vi "daqtest.vi"() -> ()   [LabVIEW 2020]
uses:
  <vilib>/DAQmx/write.llb/DAQmx Write (Analog DBL 1Chan 1Samp).vi
  <vilib>/DAQmx/write.llb/DAQmx Write (Digital Bool 1Line 1Point).vi
  <vilib>/DAQmx/create/channels.llb/DAQmx Create Channel (DO-Digital Output).vi
  <vilib>/DAQmx/miscellaneous.llb/DAQmx Fill In Error Info.vi
  <vilib>/DAQmx/create/channels.llb/DAQmx Create Channel (AO-Voltage-Basic).vi
panel:
  in  "Blanking channel":tag="Dev1/ao0"
  in  "stop":bool
  in  "physical channels 4":tag
  in  "physical channels 2":tag
  in  "physical channels":tag
  in  "Laser Channel 3":tag
  in  "Vmode":dbl=5.0 min=0.0 max=5.0
  in  "Digital Blanking Channel":tag="Dev1/port0/line4"
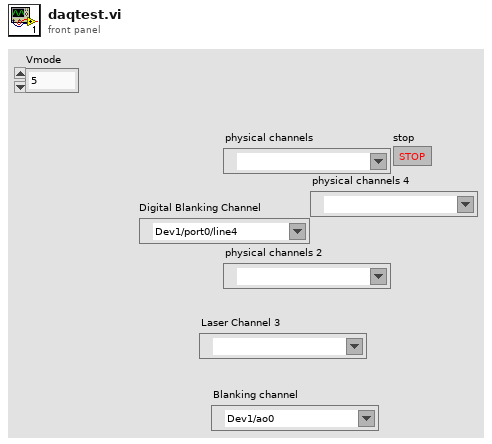
[diagram p1: front panel]
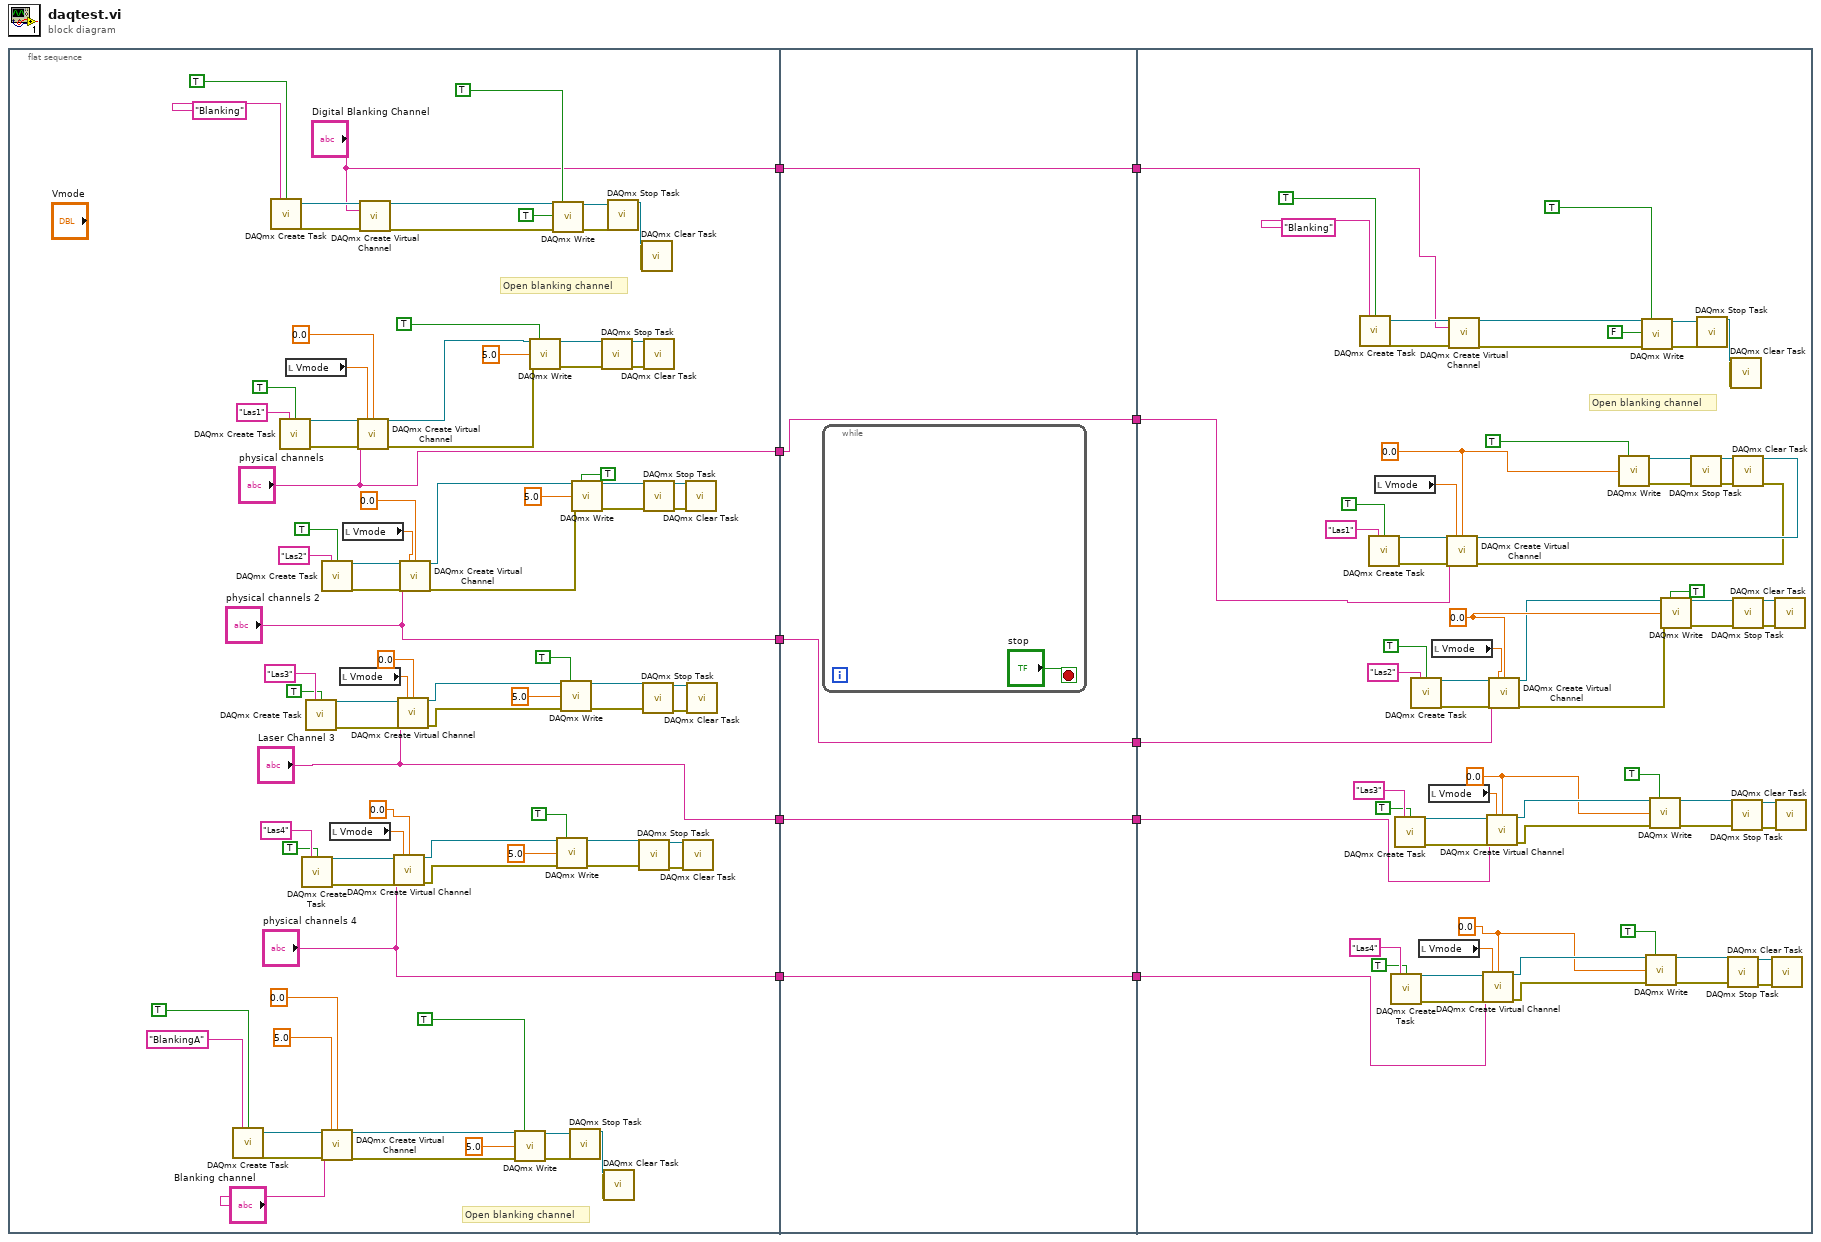
[diagram p0: block diagram]
diagram:
  n1 = flat-sequence {
    tunnel: ["Laser Channel 3"] -> w9
    tunnel: ["physical channels 4"] -> w7
    tunnel: ["physical channels 2"] -> w6
    tunnel: ["physical channels"] -> w3
    tunnel: ["Digital Blanking Channel"] -> w2
    tunnel: [w103] -> w10
    tunnel: w9 -> [w103]
    tunnel: [w102] -> w8
    tunnel: w7 -> [w102]
    tunnel: w6 -> [w101]
    tunnel: [w101] -> w5
    tunnel: [w100] -> w4
    tunnel: w3 -> [w100]
    tunnel: w2 -> [w99]
    tunnel: [w99] -> w1
    tunnel: w10 -> [w109]
    tunnel: w8 -> [w108]
    tunnel: w5 -> [w107]
    tunnel: w4 -> [w106]
    tunnel: w1 -> [w105]
    frame #0 {
      # "Open blanking channel"
      # "Open blanking channel"
      n2 = call <vilib>:"DAQmx Create Task.vi"("new task name"="BlankingA", "auto cleanup"=TRUE) -> ("task out"=w22:refnum<k21>, "error out"=w23:errorcluster)  [unwired: 12 in]
      n3 = call <vilib>:"DAQmx Create Task.vi"("new task name"="Blanking", "auto cleanup"=TRUE) -> ("task out"=w95:refnum<k21>, "error out"=w96:errorcluster)  [unwired: 12 in]
      n4 = call <vilib>:"DAQmx Create Task.vi"("new task name"="Las1", "auto cleanup"=TRUE) -> ("task out"=w68:refnum<k21>, "error out"=w67:errorcluster)  [unwired: 12 in]
      n5 = local read "Vmode"() -> (w64:dbl)
      n6 = call <vilib>:"DAQmx Create Task.vi"("new task name"="Las4", "auto cleanup"=TRUE) -> ("task out"=w48:refnum<k21>, "error out"=w46:errorcluster)  [unwired: 12 in]
      n7 = call <vilib>:"DAQmx Create Task.vi"("new task name"="Las3", "auto cleanup"=TRUE) -> ("task out"=w61:refnum<k21>, "error out"=w58:errorcluster)  [unwired: 12 in]
      n8 = call <vilib>:"DAQmx Create Task.vi"("new task name"="Las2", "auto cleanup"=TRUE) -> ("task out"=w80:refnum<k21>, "error out"=w79:errorcluster)  [unwired: 12 in]
      n9 = call-poly <vilib>:"DAQmx Create Virtual Channel.vi"("task in"=w22, "maximum value"=5.0, "minimum value"=0.0, "physical channels"="Blanking channel", "error in"=w23) -> ("task out"=w21:refnum<k21>, "error out"=w20:errorcluster)  [unwired: 9 in]
      n10 = local read "Vmode"() -> (w38:dbl)
      n11 = local read "Vmode"() -> (w60:dbl)
      n12 = local read "Vmode"() -> (w63:dbl)
      n13 = call-poly <vilib>:"DAQmx Create Virtual Channel.vi"("task in"=w68, "maximum value"=w64, "minimum value"=0.0 ("data"), "physical channels"="physical channels", "error in"=w67) -> ("task out"=w27:refnum<k21>, "error out"=w26:errorcluster)  [unwired: 9 in]
      n14 = call-poly <vilib>:"DAQmx Create Virtual Channel.vi"("task in"=w95, "lines"="Digital Blanking Channel", "error in"=w96) -> ("task out"=w94:refnum<k21>, "error out"=w93:errorcluster)  [unwired: 11 in]
      n15 = call-poly <vilib>:"DAQmx Create Virtual Channel.vi"("task in"=w48, "maximum value"=w38, "minimum value"=0.0, "physical channels"="physical channels 4", "error in"=w46) -> ("task out"=w45:refnum<k21>, "error out"=w44:errorcluster)  [unwired: 9 in]
      n16 = call-poly <vilib>:"DAQmx Create Virtual Channel.vi"("task in"=w61, "maximum value"=w60, "minimum value"=0.0, "physical channels"="Laser Channel 3", "error in"=w58) -> ("task out"=w57:refnum<k21>, "error out"=w56:errorcluster)  [unwired: 9 in]
      n17 = call-poly <vilib>:"DAQmx Create Virtual Channel.vi"("task in"=w80, "maximum value"=w63, "minimum value"=0.0 ("data"), "physical channels"="physical channels 2", "error in"=w79) -> ("task out"=w78:refnum<k21>, "error out"=w77:errorcluster)  [unwired: 9 in]
      n18 = call-poly <vilib>:"DAQmx Write.vi"("task/channels in"=w21, "auto start"=TRUE, "data"=5.0, "error in"=w20) -> ("task out"=w25:refnum<k21>, "error out"=w24:errorcluster)  [unwired: 9 in, 1 out]
      n19 = call-poly <vilib>:"DAQmx Write.vi"("task/channels in"=w27, "auto start"=TRUE ("auto cleanup"), "data"=5.0, "error in"=w26) -> ("task out"=w70:refnum<k21>, "error out"=w69:errorcluster)  [unwired: 9 in, 1 out]
      n20 = call-poly <vilib>:"DAQmx Write.vi"("task/channels in"=w94, "auto start"=TRUE, "data"=TRUE, "error in"=w93) -> ("task out"=w98:refnum<k21>, "error out"=w97:errorcluster)  [unwired: 9 in, 1 out]
      n21 = call-poly <vilib>:"DAQmx Write.vi"("task/channels in"=w45, "auto start"=TRUE, "data"=5.0, "error in"=w44) -> ("task out"=w40:refnum<k21>, "error out"=w39:errorcluster)  [unwired: 9 in, 1 out]
      n22 = call-poly <vilib>:"DAQmx Write.vi"("task/channels in"=w57, "auto start"=TRUE, "data"=5.0, "error in"=w56) -> ("task out"=w51:refnum<k21>, "error out"=w50:errorcluster)  [unwired: 9 in, 1 out]
      n23 = call <vilib>:"DAQmx Stop Task.vi"("task/channels in"=w25, "error in"=w24) -> ("task out"=w18:refnum<k21>, "error out"=w17:errorcluster)  [unwired: 12 in]
      n24 = call-poly <vilib>:"DAQmx Write.vi"("task/channels in"=w78, "auto start"=TRUE ("auto cleanup"), "data"=5.0, "error in"=w77) -> ("task out"=w82:refnum<k21>, "error out"=w81:errorcluster)  [unwired: 9 in, 1 out]
      n25 = call <vilib>:"DAQmx Stop Task.vi"("task/channels in"=w70, "error in"=w69) -> ("task out"=w66:refnum<k21>, "error out"=w65:errorcluster)  [unwired: 12 in]
      n26 = call <vilib>:"DAQmx Clear Task.vi"("task in"=w18, "error in"=w17) -> ()  [unwired: 13 in, 1 out]
      n27 = call <vilib>:"DAQmx Stop Task.vi"("task/channels in"=w98, "error in"=w97) -> ("task out"=w91:refnum<k21>, "error out"=w90:errorcluster)  [unwired: 12 in]
      n28 = call <vilib>:"DAQmx Stop Task.vi"("task/channels in"=w40, "error in"=w39) -> ("task out"=w42:refnum<k21>, "error out"=w41:errorcluster)  [unwired: 12 in]
      n29 = call <vilib>:"DAQmx Clear Task.vi"("task in"=w91, "error in"=w90) -> ()  [unwired: 13 in, 1 out]
      n30 = call <vilib>:"DAQmx Stop Task.vi"("task/channels in"=w51, "error in"=w50) -> ("task out"=w53:refnum<k21>, "error out"=w52:errorcluster)  [unwired: 12 in]
      n31 = call <vilib>:"DAQmx Clear Task.vi"("task in"=w66, "error in"=w65) -> ()  [unwired: 13 in, 1 out]
      n32 = call <vilib>:"DAQmx Stop Task.vi"("task/channels in"=w82, "error in"=w81) -> ("task out"=w76:refnum<k21>, "error out"=w75:errorcluster)  [unwired: 12 in]
      n33 = call <vilib>:"DAQmx Clear Task.vi"("task in"=w42, "error in"=w41) -> ()  [unwired: 13 in, 1 out]
      n34 = call <vilib>:"DAQmx Clear Task.vi"("task in"=w76, "error in"=w75) -> ()  [unwired: 13 in, 1 out]
      n35 = call <vilib>:"DAQmx Clear Task.vi"("task in"=w53, "error in"=w52) -> ()  [unwired: 13 in, 1 out]
    }
    frame #1 {
      n36 = while {
        stop <- "stop" stop-if-true
      }
    }
    frame #2 {
      w110 = 0.0 ("minimum value")
      w127 = 0.0 ("minimum value")
      w161 = 0.0 ("data")
      w149 = 0.0 ("data")
      # "Open blanking channel"
      n37 = call <vilib>:"DAQmx Create Task.vi"("new task name"="Blanking", "auto cleanup"=TRUE) -> ("task out"=w170:refnum<k21>, "error out"=w171:errorcluster)  [unwired: 12 in]
      n38 = call <vilib>:"DAQmx Create Task.vi"("new task name"="Las1", "auto cleanup"=TRUE) -> ("task out"=w143:refnum<k21>, "error out"=w142:errorcluster)  [unwired: 12 in]
      n39 = local read "Vmode"() -> (w137:dbl)
      n40 = call <vilib>:"DAQmx Create Task.vi"("new task name"="Las4", "auto cleanup"=TRUE) -> ("task out"=w121:refnum<k21>, "error out"=w119:errorcluster)  [unwired: 12 in]
      n41 = call <vilib>:"DAQmx Create Task.vi"("new task name"="Las3", "auto cleanup"=TRUE) -> ("task out"=w134:refnum<k21>, "error out"=w131:errorcluster)  [unwired: 12 in]
      n42 = call <vilib>:"DAQmx Create Task.vi"("new task name"="Las2", "auto cleanup"=TRUE) -> ("task out"=w155:refnum<k21>, "error out"=w154:errorcluster)  [unwired: 12 in]
      n43 = local read "Vmode"() -> (w111:dbl)
      n44 = local read "Vmode"() -> (w133:dbl)
      n45 = local read "Vmode"() -> (w136:dbl)
      n46 = call-poly <vilib>:"DAQmx Create Virtual Channel.vi"("task in"=w143, "maximum value"=w137, "minimum value"=w149, "physical channels"=w106, "error in"=w142) -> ("task out"=w141:refnum<k21>, "error out"=w140:errorcluster)  [unwired: 9 in]
      n47 = call-poly <vilib>:"DAQmx Create Virtual Channel.vi"("task in"=w170, "lines"=w105, "error in"=w171) -> ("task out"=w169:refnum<k21>, "error out"=w168:errorcluster)  [unwired: 11 in]
      n48 = call-poly <vilib>:"DAQmx Create Virtual Channel.vi"("task in"=w121, "maximum value"=w111, "minimum value"=w110, "physical channels"=w108, "error in"=w119) -> ("task out"=w118:refnum<k21>, "error out"=w117:errorcluster)  [unwired: 9 in]
      n49 = call-poly <vilib>:"DAQmx Create Virtual Channel.vi"("task in"=w134, "maximum value"=w133, "minimum value"=w127, "physical channels"=w109, "error in"=w131) -> ("task out"=w130:refnum<k21>, "error out"=w129:errorcluster)  [unwired: 9 in]
      n50 = call-poly <vilib>:"DAQmx Create Virtual Channel.vi"("task in"=w155, "maximum value"=w136, "minimum value"=w161, "physical channels"=w107, "error in"=w154) -> ("task out"=w153:refnum<k21>, "error out"=w152:errorcluster)  [unwired: 9 in]
      n51 = call-poly <vilib>:"DAQmx Write.vi"("task/channels in"=w141, "auto start"=TRUE ("auto cleanup"), "data"=w149, "error in"=w140) -> ("task out"=w145:refnum<k21>, "error out"=w144:errorcluster)  [unwired: 9 in, 1 out]
      n52 = call-poly <vilib>:"DAQmx Write.vi"("task/channels in"=w169, "auto start"=TRUE, "data"=FALSE, "error in"=w168) -> ("task out"=w173:refnum<k21>, "error out"=w172:errorcluster)  [unwired: 9 in, 1 out]
      n53 = call-poly <vilib>:"DAQmx Write.vi"("task/channels in"=w118, "auto start"=TRUE, "data"=w110, "error in"=w117) -> ("task out"=w113:refnum<k21>, "error out"=w112:errorcluster)  [unwired: 9 in, 1 out]
      n54 = call-poly <vilib>:"DAQmx Write.vi"("task/channels in"=w130, "auto start"=TRUE, "data"=w127, "error in"=w129) -> ("task out"=w124:refnum<k21>, "error out"=w123:errorcluster)  [unwired: 9 in, 1 out]
      n55 = call-poly <vilib>:"DAQmx Write.vi"("task/channels in"=w153, "auto start"=TRUE ("auto cleanup"), "data"=w161, "error in"=w152) -> ("task out"=w157:refnum<k21>, "error out"=w156:errorcluster)  [unwired: 9 in, 1 out]
      n56 = call <vilib>:"DAQmx Stop Task.vi"("task/channels in"=w145, "error in"=w144) -> ("task out"=w139:refnum<k21>, "error out"=w138:errorcluster)  [unwired: 12 in]
      n57 = call <vilib>:"DAQmx Stop Task.vi"("task/channels in"=w173, "error in"=w172) -> ("task out"=w166:refnum<k21>, "error out"=w165:errorcluster)  [unwired: 12 in]
      n58 = call <vilib>:"DAQmx Stop Task.vi"("task/channels in"=w113, "error in"=w112) -> ("task out"=w115:refnum<k21>, "error out"=w114:errorcluster)  [unwired: 12 in]
      n59 = call <vilib>:"DAQmx Clear Task.vi"("task in"=w166, "error in"=w165) -> ()  [unwired: 13 in, 1 out]
      n60 = call <vilib>:"DAQmx Stop Task.vi"("task/channels in"=w124, "error in"=w123) -> ("task out"=w126:refnum<k21>, "error out"=w125:errorcluster)  [unwired: 12 in]
      n61 = call <vilib>:"DAQmx Clear Task.vi"("task in"=w139, "error in"=w138) -> ()  [unwired: 13 in, 1 out]
      n62 = call <vilib>:"DAQmx Stop Task.vi"("task/channels in"=w157, "error in"=w156) -> ("task out"=w151:refnum<k21>, "error out"=w150:errorcluster)  [unwired: 12 in]
      n63 = call <vilib>:"DAQmx Clear Task.vi"("task in"=w115, "error in"=w114) -> ()  [unwired: 13 in, 1 out]
      n64 = call <vilib>:"DAQmx Clear Task.vi"("task in"=w151, "error in"=w150) -> ()  [unwired: 13 in, 1 out]
      n65 = call <vilib>:"DAQmx Clear Task.vi"("task in"=w126, "error in"=w125) -> ()  [unwired: 13 in, 1 out]
    }
  }
